vi "FGVCalibrations.vi"(7 "Enum":T2, 8 "error in":errorcluster, 10 "calibIn":T1 {"calibParameters"."HV gain"."HV gain X" format="%#.0f"; "calibParameters"."HV gain"."HV gain Y" format="%#.0f"; "calibParameters"."HV gain"."HV gain Z" format="%#.0f"; "calibParameters"."Range"."Range X" format="%#.2pm"; "calibParameters"."Range"."Range Y" format="%#.2pm"; "calibParameters"."Range"."Range Z" format="%#.2pm"; "calibParameters"."Sensitivity"."Sens X" format="%#.2pm/V"; "calibParameters"."Sensitivity"."Sens Y" format="%#.2pm/V"; "calibParameters"."Sensitivity"."Sens Z" format="%#.2pm/V"}) -> (0 "error out":errorcluster, 2 "calibOut":T1 {"calibParameters"."HV gain"."HV gain X" format="%#.0f"; "calibParameters"."HV gain"."HV gain Y" format="%#.0f"; "calibParameters"."HV gain"."HV gain Z" format="%#.0f"; "calibParameters"."Range"."Range X" format="%#.2pm"; "calibParameters"."Range"."Range Y" format="%#.2pm"; "calibParameters"."Range"."Range Z" format="%#.2pm"; "calibParameters"."Sensitivity"."Sens X" format="%#.2pm/V"; "calibParameters"."Sensitivity"."Sens Y" format="%#.2pm/V"; "calibParameters"."Sensitivity"."Sens Z" format="%#.2pm/V"})   [LabVIEW 2016]
uses:
  controls/Enum.ctl
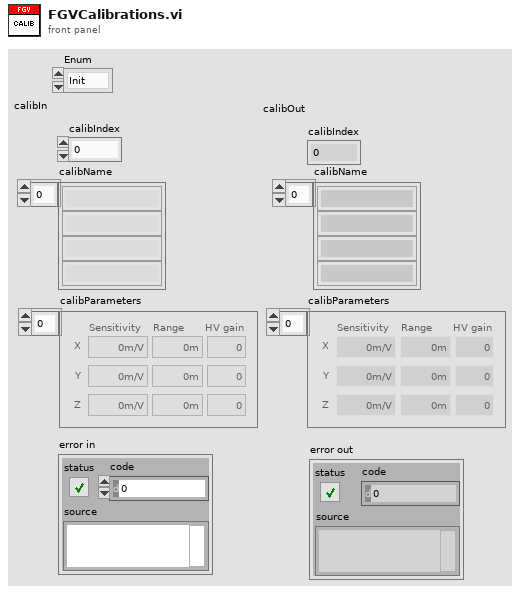
[diagram p1: front panel]
types:
  T1 = cluster{"calibName":string[], "calibParameters":cluster{"Sensitivity":cluster{"Sens X":dbl, "Sens Y":dbl, "Sens Z":dbl}, "Range":cluster{"Range X":dbl, "Range Y":dbl, "Range Z":dbl}, "HV gain":cluster{"HV gain X":dbl, "HV gain Y":dbl, "HV gain Z":dbl}}[], "calibIndex":i32}
  T2 = typedef "Enum.ctl" = enum16{"Init", "Read", "Write"}
  T3 = cluster{"Sensitivity":cluster{"Sens Z":dbl, "Sens Y":dbl, "Sens X":dbl}, "Range":cluster{"Range Z":dbl, "Range Y":dbl, "Range X":dbl}, "HV gain":cluster{"HV gain Z":i32, "HV gain Y":i32, "HV gain X":i32}}
  T4 = cluster{"Sensitivity":cluster{"Sens Z":dbl, "Sens Y":dbl, "Sens X":dbl}, "Range":cluster{"Range Z":dbl, "Range Y":dbl, "Range X":dbl}, "HV gain":cluster{"HV gain Z":i32, "HV gain Y":i32, "HV gain X":i32}}[]
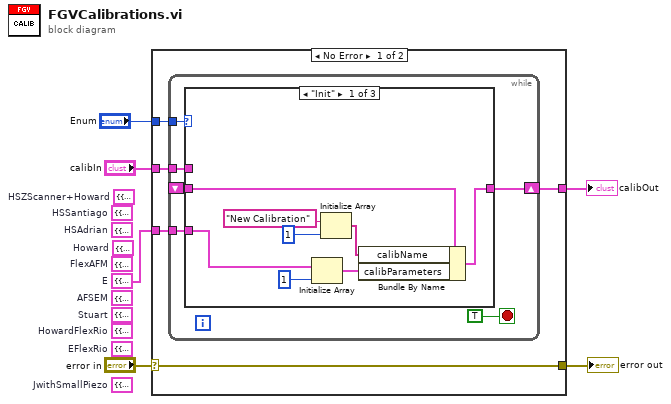
[diagram p0: block diagram]
diagram:
  (unwired) T3 {"Sensitivity"={"Sens Z"=6.5e-07, "Sens Y"=6.6e-07, "Sens X"=2e-07}, "Range"={"Range Z"=0.00013, "Range Y"=0.000132, "Range X"=2e-06}, "HV gain"={"HV gain Z"=20, "HV gain Y"=20, "HV gain X"=20}}  # JwithSmallPiezo
  (unwired) T3 {"Sensitivity"={"Sens Z"=6.5e-07, "Sens Y"=6.6e-07, "Sens X"=2.5e-07}, "Range"={"Range Z"=0.00013, "Range Y"=0.000132, "Range X"=1.1803e-06}, "HV gain"={"HV gain Z"=20, "HV gain Y"=20, "HV gain X"=20}}  # HSZScanner+Howard
  (unwired) T3 {"Sensitivity"={"Sens Z"=2.8e-08, "Sens Y"=3.2e-08, "Sens X"=8.7}, "Range"={"Range Z"=8.63309e-06, "Range Y"=1.00236e-05, "Range X"=1.0457e-06}, "HV gain"={"HV gain Z"=20, "HV gain Y"=20, "HV gain X"=20}}  # EFlexRio
  (unwired) T3 {"Sensitivity"={"Sens Z"=6.5e-07, "Sens Y"=6.6e-07, "Sens X"=2.5e-07}, "Range"={"Range Z"=0.00013, "Range Y"=0.000132, "Range X"=4.33e-06}, "HV gain"={"HV gain Z"=20, "HV gain Y"=20, "HV gain X"=20}}  # Howard
  (unwired) T3 {"Sensitivity"={"Sens Z"=2.66e-08, "Sens Y"=2.66e-08, "Sens X"=3e-08}, "Range"={"Range Z"=5.5e-05, "Range Y"=5.5e-05, "Range X"=2.3e-05}, "HV gain"={"HV gain Z"=1, "HV gain Y"=1, "HV gain X"=1}}  # Stuart
  w1 = T3 {"Sensitivity"={"Sens Z"=2.8e-08, "Sens Y"=3.2e-08, "Sens X"=8.7}, "Range"={"Range Z"=1.2e-05, "Range Y"=1.2e-05, "Range X"=3.5e-06}, "HV gain"={"HV gain Z"=20, "HV gain Y"=20, "HV gain X"=20}}  # E
  (unwired) T3 {"Sensitivity"={"Sens Z"=1e-05, "Sens Y"=1e-05, "Sens X"=1e-06}, "Range"={"Range Z"=0.0001, "Range Y"=0.0001, "Range X"=1e-05}, "HV gain"={"HV gain Z"=1, "HV gain Y"=1, "HV gain X"=1}}  # FlexAFM
  (unwired) T3 {"Sensitivity"={"Sens Z"=6.5e-07, "Sens Y"=6.6e-07, "Sens X"=2.5e-07}, "Range"={"Range Z"=0.00010169, "Range Y"=0.00013107, "Range X"=7e-06}, "HV gain"={"HV gain Z"=20, "HV gain Y"=20, "HV gain X"=20}}  # HowardFlexRio
  (unwired) T3 {"Sensitivity"={"Sens Z"=2.66e-08, "Sens Y"=2.66e-08, "Sens X"=3e-08}, "Range"={"Range Z"=1.6e-06, "Range Y"=1.6e-06, "Range X"=1.8e-06}, "HV gain"={"HV gain Z"=6, "HV gain Y"=6, "HV gain X"=6}}  # HSAdrian
  (unwired) T3 {"Sensitivity"={"Sens Z"=2.66e-08, "Sens Y"=2.66e-08, "Sens X"=3e-08}, "Range"={"Range Z"=3e-05, "Range Y"=3e-05, "Range X"=1e-05}, "HV gain"={"HV gain Z"=1, "HV gain Y"=1, "HV gain X"=1}}  # AFSEM
  (unwired) T3 {"Sensitivity"={"Sens Z"=2.3e-09, "Sens Y"=2.3e-09, "Sens X"=3.33e-09}, "Range"={"Range Z"=1.4e-06, "Range Y"=1.4e-06, "Range X"=2e-06}, "HV gain"={"HV gain Z"=60, "HV gain Y"=60, "HV gain X"=60}}  # HSSantiago
  n1 = case shown="No Error" "error in" {
    selector: "error in" -> [w10 w29]
    tunnel: "Enum" -> [w11 _]
    tunnel: [w10 w29] -> w5
    tunnel: "calibIn" -> [w9 w28]
    tunnel: [w8 w28] -> w3
    tunnel: w1 -> [w7 _]
    frame No Error {
      n2 = while {
        tunnel: w11 -> [w16]
        tunnel: w9 -> [w15]
        shift-right: [w14] -> w8
        shift-left: _ -> [w13]
        tunnel: w7 -> [w12]
        stop <- TRUE stop-if-true
        n3 = case shown="\"Init\"" w16 {
          tunnel: w15 -> [_ _ w27]
          tunnel: [w25 w26 w27] -> w14
          tunnel: w13 -> [w24 w26 _]
          tunnel: w12 -> [w18 _ _]
          frame "Init" {
            n4 = Initialize Array(w18, 1 ("dimension size")) -> (w19:T4)
            n5 = Initialize Array("New Calibration", 1 ("dimension size")) -> (w21:string[])
            n6 = Bundle By Name(cluster=w24, "calibName"=w21, "calibParameters"=w19) -> (w25:T1)
          }
          frame "Read", Default {
          }
          frame "Write" {
          }
        }
      }
    }
    frame Error {
    }
  }
  "error out" <- w5
  "calibOut" <- w3
